vi "Clear Table.vi"(8 "error in (no error)":errorcluster, 11 "Cyclic Table in":refnum<class "Cyclic Table.lvclass">) -> (0 "error out":errorcluster, 3 "Cyclic Table out":refnum<class "Cyclic Table.lvclass">)   [LabVIEW 2024, in "Cyclic Table.lvclass"]
doc: "Clear all entries in table."
uses:
  Cyclic Table.lvclass
  Cyclic Table.lvclass/Cyclic Table.ctl
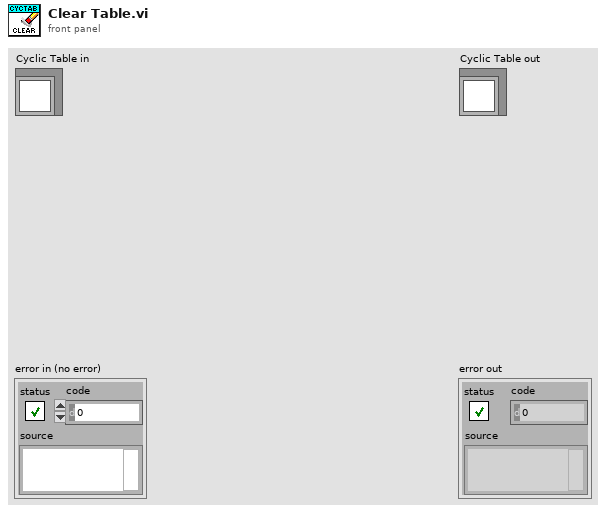
[diagram p1: front panel]
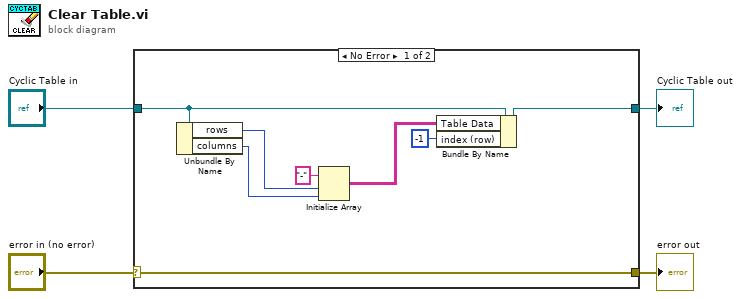
[diagram p0: block diagram]
diagram:
  n1 = case shown="No Error" "error in (no error)" {
    selector: "error in (no error)" -> [w12 w14]
    tunnel: [w12 w14] -> w3
    tunnel: [w11 w13] -> w1
    tunnel: "Cyclic Table in" -> [w10 w13]
    frame No Error {
      n2 = Unbundle By Name(w10) -> ("rows"=w8:i32, "columns"=w7:i32)
      n3 = Initialize Array("-" ("Message Class"), w8, w7) -> (w6:string[][])
      n4 = Bundle By Name(cluster=w10, "Table Data"=w6, "index (row)"=-1) -> (w11:refnum<class "Cyclic Table.lvclass">)
    }
    frame Error {
    }
  }
  "error out" <- w3
  "Cyclic Table out" <- w1
